vi "Get Handles for Scan Devices.vi"(2 "Old Device Names":string[](array[string]), 3 "All Handles In":i32[](array[numeric]), 4 "New Device Names":string[](array[string])) -> (0 "All Handles Out":i32[](array[numeric]), 1 "# handles":i32)   [LabVIEW 2018, in "Powermeter_library.lvlib"]
uses:
  Powermeter_library.lvlib
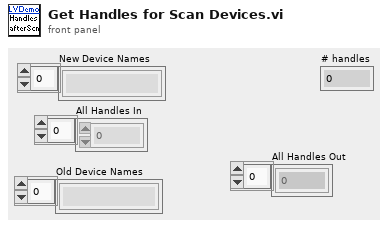
[diagram p1: front panel]
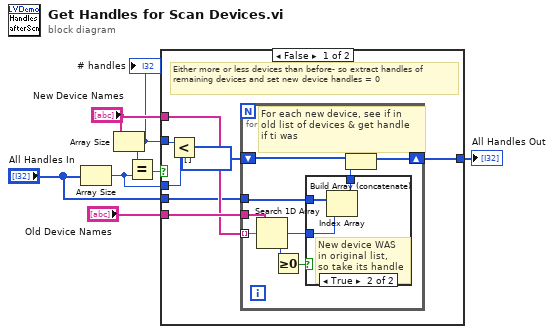
[diagram p0: block diagram]
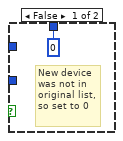
[diagram p2: hidden frame]
diagram:
  n1 = Array Size(array="All Handles In") -> (size(s)=w5:i32)
  n2 = Array Size(array="New Device Names") -> (size(s)=w2:i32)
  "# handles" <- w2
  n3 = Equal?(x=w2, y=w5) -> (x = y?=w4:bool)
  n4 = case shown="False" w4 {
    tunnel: [w9 w27] -> w1
    tunnel: w2 -> [w14 _]
    tunnel: "All Handles In" -> [w10 w27]
    tunnel: w5 -> [w13 _]
    tunnel: "Old Device Names" -> [w12 _]
    tunnel: "New Device Names" -> [w11 _]
    frame False {
      # "Either more or less devices than before- so extract handles of remaining devices and set new device handles = 0"
      n5 = Less?(x=w14, y=w13) -> ()  [unwired: 1 out]
      n6 = for {
        tunnel: w11 -> [w22] mode=indexing
        tunnel: w12 -> [w21]
        tunnel: w10 -> [w19]
        shift-right: [w16] -> w9
        shift-left: i32[] [] -> [w17]
        # "For each new device, see if in\nold list of devices & get handle\nif ti was"
        n7 = Search 1D Array(1D array=w21, element=w22) -> (index of element=w18:i32)  [unwired: 1 out]
        n8 = Greater Or Equal To 0?(x=w18) -> (x >= 0?=w20:bool)
        n9 = case shown="True" w20 {
          tunnel: w19 -> [_ w26]
          tunnel: w18 -> [_ w25]
          tunnel: [0 ("Numeric") w24] -> w15
          frame False {
            # "New device\nwas not in \noriginal list,\nso set to 0"
          }
          frame True {
            # "New device WAS\nin original list,\nso take its handle"
            n10 = Index Array(array=w26, index=w25) -> (element=w24:i32)
          }
        }
        n11 = Build Array (concatenate)(w17, w15) -> (w16:i32[])
      }
    }
    frame True {
      # "No change in # of devices, so just use old handles"
    }
  }
  "All Handles Out" <- w1
